vi "7.vi"() -> ()   [LabVIEW 2023]
panel:
  out "Waveform Chart":cluster{dbl, "xB":dbl}(graph)
  in  "Stop Button":bool
  in  "yB":u16(slide) scale=0.0..600.0
  in  "Turatie":u8(slide) scale=10.0..60.0
  in  "L2":u8(slide) scale=0.0..200.0
  in  "L1":u8(slide) scale=0.0..100.0
  in  "xO":u16(slide) scale=0.0..900.0
  in  "yO":u16(slide) scale=0.0..600.0
  out "2D Picture":picture
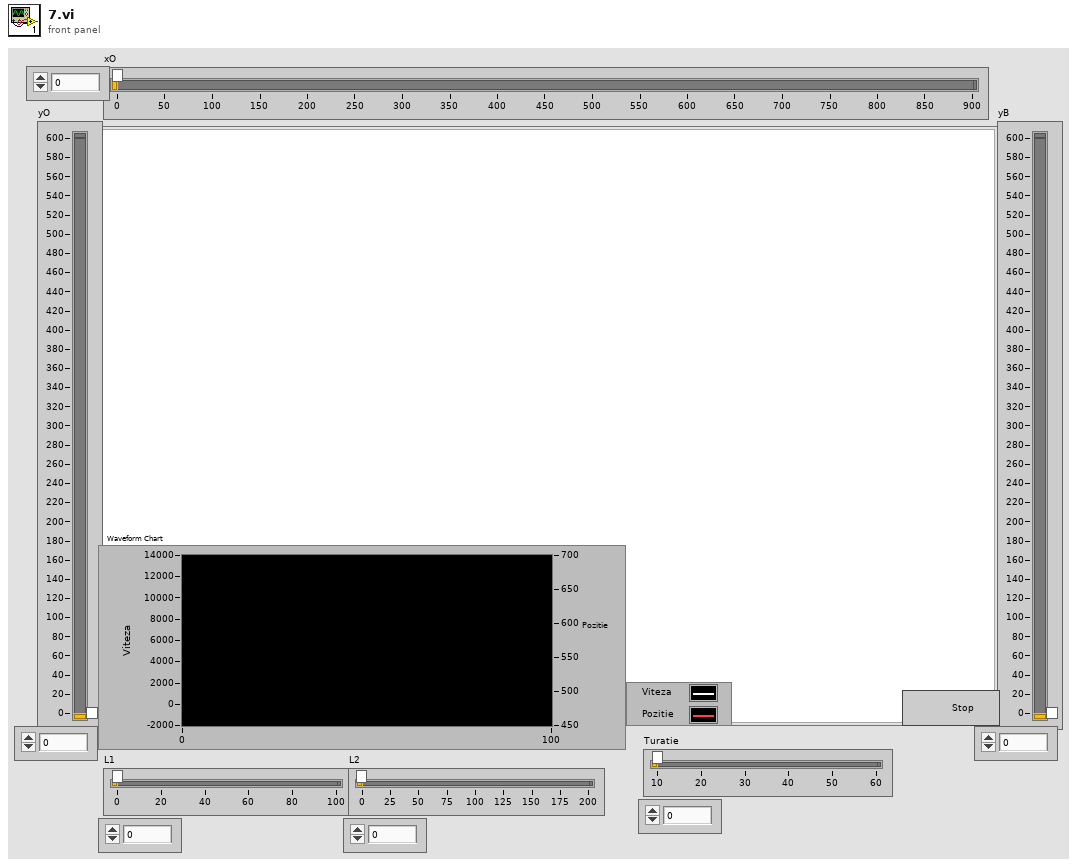
[diagram p1: front panel]
types:
  T1 = cluster{"Width":u16, "Style":enum32{"Solid", "Dash", "Dot", "DashDot", "DashDotDot"}}
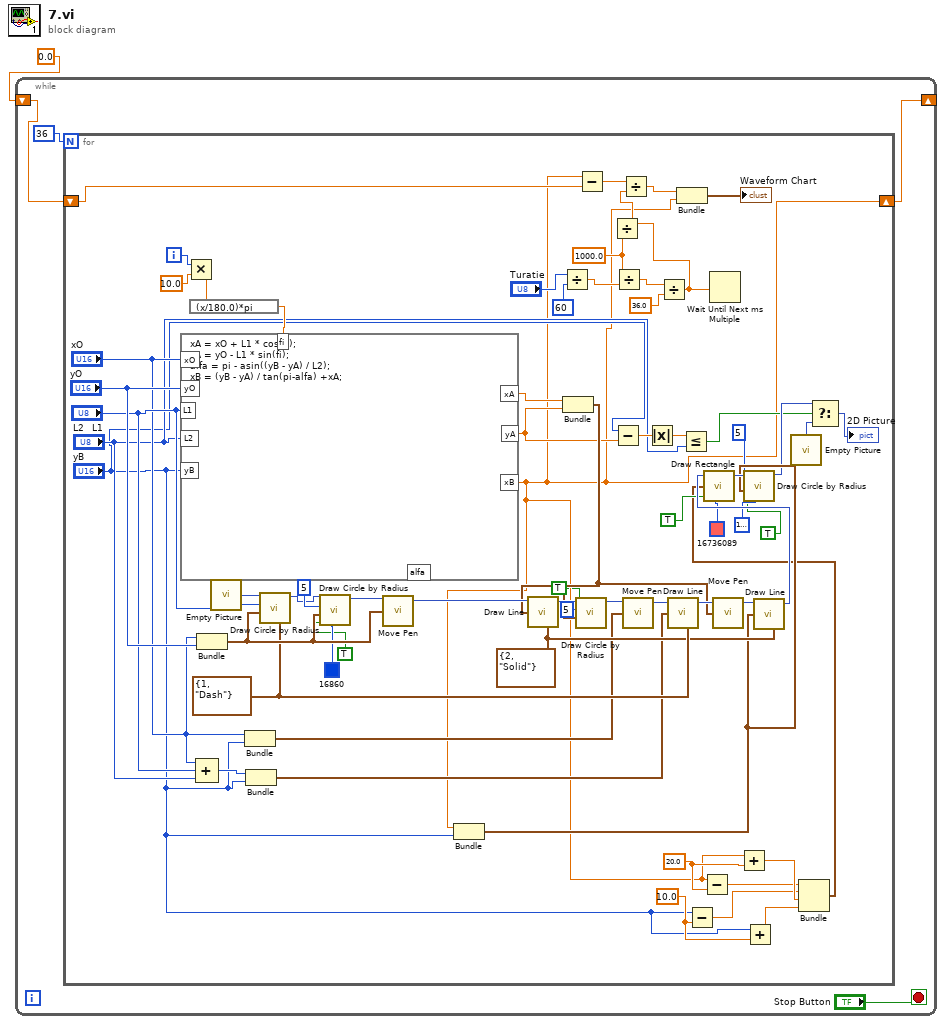
[diagram p0: block diagram]
diagram:
  n1 = while {
    shift-right: [w2] -> _
    shift-left: 0.0 -> [w3]
    stop <- "Stop Button" stop-if-true
    n2 = for {
      N: 36 -> [_]
      shift-right: [w8] -> w2
      shift-left: w3 -> [w9]
      i -> [w71]
      w14 = 1000.0
      w32 = 10.0
      w34 = 20.0
      w50 = T1 {"Width"=2, "Style"=enum."Solid"} ("pen")
      w51 = T1 {"Width"=1, "Style"=enum."Dash"} ("pen")
      n3 = Multiply(x=w71, y=10.0) -> (x*y=w70:dbl)
      n4 = expression code="(x/180.0)*pi"(w70) -> (w68:dbl)
      n5 = formula code="xA = xO + L1 * cos(fi);\nyA = yO - L1 * sin(fi);\nalfa = pi - asin((yB - yA) / L2);\nxB = (yB - yA) / tan(pi-alfa) +xA;"("xO"="xO", "yO"="yO", "L1"="L1", "L2"="L2", "yB"="yB", "fi"=w68) -> ("xA"=w67:dbl, "yA"=w22:dbl, "xB"=w8:dbl)  [unwired: 1 out]
      n6 = Compound Arithmetic op=ADD("xO", "L1", "L2") -> (w48:u16)
      n7 = Bundle("xO"="xO", "yO"="yO") -> (w63:cluster{"xO":u16, "yO":u16})  [unwired: 1 in]
      n8 = call "Empty Picture"() -> ("empty picture"=w65:picture)
      n9 = Bundle("xO"="xO", "yB"="yB") -> (w46:cluster{"xO":u16, "yB ":u16})  [unwired: 1 in]
      n10 = Bundle(w48, "yB"="yB") -> (w45:cluster{u16, "yB ":u16})  [unwired: 1 in]
      n11 = call <vilib>:"Draw Circle by Radius.vi"("pen"=w51, "pixel center"=w63, "radius"="L1", "picture"=w65) -> ("new picture"=w60:picture)  [unwired: 7 in]
      n12 = call <vilib>:"Draw Circle by Radius.vi"("color(black)"=u32 16860, "fill?(F)"=TRUE, "pixel center"=w63, "radius"=5, "picture"=w60) -> ("new picture"=w59:picture)  [unwired: 6 in]
      n13 = call <vilib>:"Move Pen.vi"("new position"=w63, "picture"=w59) -> ("new picture"=w58:picture)  [unwired: 3 in]
      n14 = Bundle("xB"=w8, "yB"="yB") -> (w38:cluster{"xB":dbl, "yB ":u16})  [unwired: 1 in]
      n15 = Divide(x="Turatie", y=60) -> (x/y=w19:dbl)
      n16 = Bundle("xA"=w67, "yA"=w22) -> (w53:cluster{"xA":dbl, "yA":dbl})  [unwired: 1 in]
      n17 = call <vilib>:"Draw Line.vi"("picture"=w58, "end point"=w53, "pen"=w50) -> ("new picture"=w57:picture)  [unwired: 6 in]
      n18 = call <vilib>:"Draw Circle by Radius.vi"("fill?(F)"=TRUE, "pixel center"=w53, "radius"=i16 5, "picture"=w57) -> ("new picture"=w56:picture)  [unwired: 7 in]
      n19 = Subtract(x=w8, y=w9) -> (x-y=w10:dbl)
      n20 = Subtract(x="yB", y=w22) -> (x-y=w26:dbl)
      n21 = Divide(x=w14, y=w19) -> (x/y=w20:dbl)
      n22 = call <vilib>:"Move Pen.vi"("new position"=w46, "picture"=w56) -> ("new picture"=w55:picture)  [unwired: 3 in]
      n23 = Absolute Value(x=w26) -> (abs(x)=w25:dbl)
      n24 = Divide(x=w20, y=36.0) -> (x/y=w13:dbl)
      n25 = Divide(x=w13, y=w14) -> (x/y=w12:dbl)
      n26 = Divide(x=w10, y=w12) -> (x/y=w11:dbl)
      n27 = call <vilib>:"Draw Line.vi"("picture"=w55, "end point"=w45, "pen"=w51) -> ("new picture"=w54:picture)  [unwired: 6 in]
      n28 = Bundle(w11, "xB"=w8) -> (→"Waveform Chart":cluster{dbl, "xB":dbl})  [unwired: 1 in]
      n29 = Less Or Equal?(x=w25, y="L2") -> (x <= y?=w24:bool)
      n30 = Subtract(x="yB", y=w32) -> (x-y=w31:dbl)
      n31 = Subtract(x=w8, y=w34) -> (x-y=w33:dbl)
      n32 = Wait Until Next ms Multiple(millisecond multiple=w13) -> ()  [unwired: 1 out]
      n33 = call <vilib>:"Move Pen.vi"("new position"=w53, "picture"=w54) -> ("new picture"=w52:picture)  [unwired: 3 in]
      n34 = Add(x=w8, y=w34) -> (x+y=w36:dbl)
      n35 = Add(x="yB", y=w32) -> (x+y=w35:dbl)
      n36 = call <vilib>:"Draw Line.vi"("picture"=w52, "end point"=w38, "pen"=w50) -> ("new picture"=w44:picture)  [unwired: 6 in]
      n37 = call "Empty Picture"() -> ("empty picture"=w28:picture)
      n38 = Bundle(w33, w31, w36, w35) -> (w30:cluster{dbl, dbl, dbl, dbl})  [unwired: 1 in]
      n39 = call <vilib>:"Draw Rectangle.vi"("picture"=w44, "rect"=w30, "fill?(F)"=TRUE, "color(black)"=u32 16736089) -> ("new picture"=w43:picture)  [unwired: 5 in]
      n40 = call <vilib>:"Draw Circle by Radius.vi"("color(black)"=u32 16777224, "fill?(F)"=TRUE, "pixel center"=w38, "radius"=5, "picture"=w43) -> ("new picture"=w29:picture)  [unwired: 6 in]
      n41 = Select(t=w29, s=w24, f=w28) -> (s? t:f=→"2D Picture":picture)
    }
  }
